vi "test_libssh2_sftp_realpath.vi"() -> ()   [LabVIEW 2013, in "libssh2_integration_tests.lvlib"]
uses:
  libssh2_integration_tests.lvlib
  <vilib>/addons/_JKI Toolkits/Caraya/classes/Test/Test.lvclass
  libssh2/libssh2.lvlib
  <vilib>/addons/_JKI Toolkits/Caraya/classes/Assert/Assert.lvclass
panel:
  out "error out":errorcluster
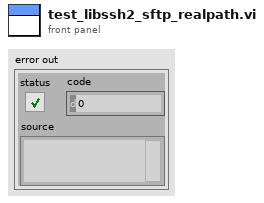
[diagram p1: front panel]
types:
  T1 = typedef "libssh2.lvlib/Session Refnum.ctl" = refnum<k1>
  T2 = typedef "libssh2.lvlib/SFTP Refnum.ctl" = refnum<k1>
  T3 = typedef "libssh2.lvlib/SFTP Handle Refnum.ctl" = refnum<k1>
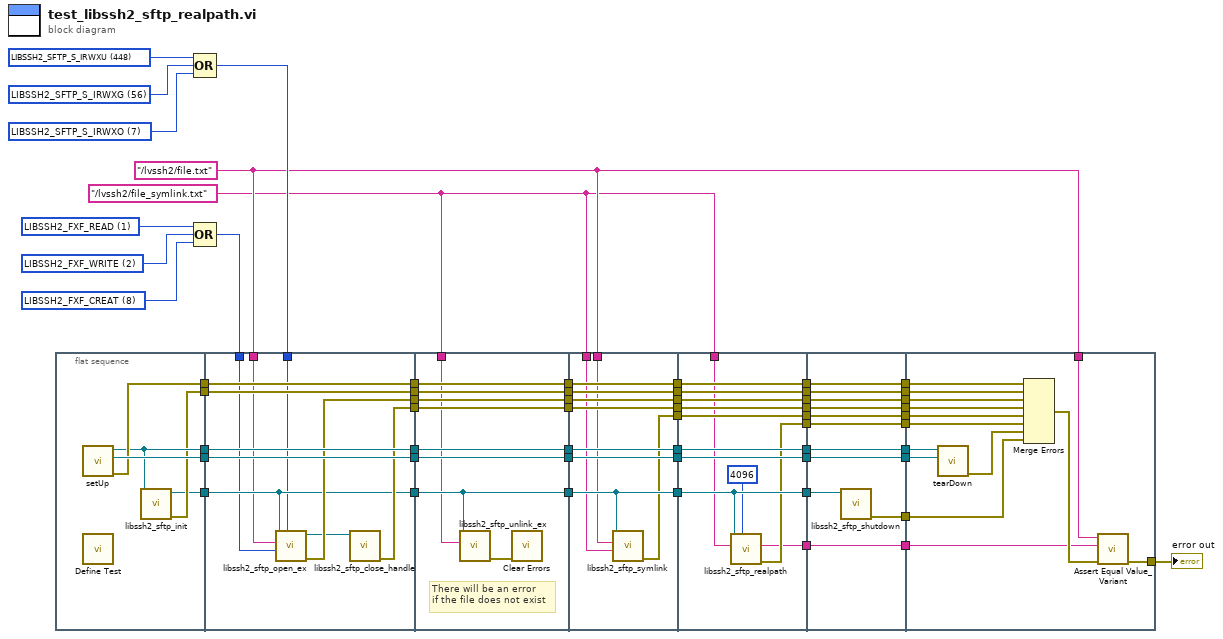
[diagram p0: block diagram]
diagram:
  w1 = "/lvssh2/file_symlink.txt" ("filename")
  w47 = u32 2 items=["LIBSSH2_FXF_READ"=1, "LIBSSH2_FXF_WRITE"=2, "LIBSSH2_FXF_APPEND"=4, "LIBSSH2_FXF_CREAT"=8, "LIBSSH2_FXF_TRUNC"=16, "LIBSSH2_FXF_EXCL"=32] ("flags")
  w48 = u32 1 items=["LIBSSH2_FXF_READ"=1, "LIBSSH2_FXF_WRITE"=2, "LIBSSH2_FXF_APPEND"=4, "LIBSSH2_FXF_CREAT"=8, "LIBSSH2_FXF_TRUNC"=16, "LIBSSH2_FXF_EXCL"=32] ("flags")
  w46 = u32 8 items=["LIBSSH2_FXF_READ"=1, "LIBSSH2_FXF_WRITE"=2, "LIBSSH2_FXF_APPEND"=4, "LIBSSH2_FXF_CREAT"=8, "LIBSSH2_FXF_TRUNC"=16, "LIBSSH2_FXF_EXCL"=32] ("flags")
  w16 = "/lvssh2/file.txt" ("filename")
  w50 = 7 items=["LIBSSH2_SFTP_S_IRWXU"=448, "LIBSSH2_SFTP_S_IRUSR"=256, "LIBSSH2_SFTP_S_IWUSR"=128, "LIBSSH2_SFTP_S_IXUSR"=64, "LIBSSH2_SFTP_S_IRWXG"=56, "LIBSSH2_SFTP_S_IRGRP"=32, "LIBSSH2_SFTP_S_IWGRP"=16, "LIBSSH2_SFTP_S_IXGRP"=8, "LIBSSH2_SFTP_S_IRWXO"=7, "LIBSSH2_SFTP_S_IROTH"=4, "LIBSSH2_SFTP_S_IWOTH"=2, "LIBSSH2_SFTP_S_IXOTH"=1] ("mode")
  w51 = 56 items=["LIBSSH2_SFTP_S_IRWXU"=448, "LIBSSH2_SFTP_S_IRUSR"=256, "LIBSSH2_SFTP_S_IWUSR"=128, "LIBSSH2_SFTP_S_IXUSR"=64, "LIBSSH2_SFTP_S_IRWXG"=56, "LIBSSH2_SFTP_S_IRGRP"=32, "LIBSSH2_SFTP_S_IWGRP"=16, "LIBSSH2_SFTP_S_IXGRP"=8, "LIBSSH2_SFTP_S_IRWXO"=7, "LIBSSH2_SFTP_S_IROTH"=4, "LIBSSH2_SFTP_S_IWOTH"=2, "LIBSSH2_SFTP_S_IXOTH"=1] ("mode")
  w52 = 448 items=["LIBSSH2_SFTP_S_IRWXU"=448, "LIBSSH2_SFTP_S_IRUSR"=256, "LIBSSH2_SFTP_S_IWUSR"=128, "LIBSSH2_SFTP_S_IXUSR"=64, "LIBSSH2_SFTP_S_IRWXG"=56, "LIBSSH2_SFTP_S_IRGRP"=32, "LIBSSH2_SFTP_S_IWGRP"=16, "LIBSSH2_SFTP_S_IXGRP"=8, "LIBSSH2_SFTP_S_IRWXO"=7, "LIBSSH2_SFTP_S_IROTH"=4, "LIBSSH2_SFTP_S_IWOTH"=2, "LIBSSH2_SFTP_S_IXOTH"=1] ("mode")
  n1 = flat-sequence {
    tunnel: [w61] -> w58
    tunnel: [w63] -> w57
    tunnel: [w62] -> w56
    tunnel: [w60] -> w54
    tunnel: [w59] -> w53
    tunnel: [w74] -> w15
    tunnel: [w73] -> w13
    tunnel: [w68] -> w11
    tunnel: [w72] -> w9
    tunnel: [w71] -> w7
    tunnel: [w70] -> w5
    tunnel: [w69] -> w3
    tunnel: w45 -> [w65]
    tunnel: w16 -> [w66]
    tunnel: w49 -> [w67]
    tunnel: w53 -> [w68]
    tunnel: w54 -> [w71]
    tunnel: w56 -> [w72]
    tunnel: w57 -> [w73]
    tunnel: w58 -> [w74]
    tunnel: w15 -> [w83]
    tunnel: [w83] -> w14
    tunnel: w13 -> [w82]
    tunnel: [w82] -> w12
    tunnel: w11 -> [w76]
    tunnel: [w76] -> w10
    tunnel: w9 -> [w81]
    tunnel: [w81] -> w8
    tunnel: w7 -> [w80]
    tunnel: [w80] -> w6
    tunnel: w5 -> [w79]
    tunnel: [w79] -> w4
    tunnel: w3 -> [w78]
    tunnel: [w78] -> w2
    tunnel: w1 -> [w75]
    tunnel: w14 -> [w93]
    tunnel: [w93] -> w36
    tunnel: w12 -> [w92]
    tunnel: [w92] -> w34
    tunnel: w10 -> [w89]
    tunnel: [w89] -> w32
    tunnel: w8 -> [w91]
    tunnel: [w91] -> w29
    tunnel: w6 -> [w90]
    tunnel: [w90] -> w27
    tunnel: w16 -> [w85]
    tunnel: w1 -> [w86]
    tunnel: w4 -> [w88]
    tunnel: [w88] -> w25
    tunnel: w2 -> [w87]
    tunnel: [w87] -> w23
    tunnel: [w84] -> w21
    tunnel: w36 -> [w105]
    tunnel: [w105] -> w35
    tunnel: w34 -> [w104]
    tunnel: [w104] -> w33
    tunnel: w32 -> [w98]
    tunnel: [w98] -> w31
    tunnel: [w95] -> w30
    tunnel: w29 -> [w103]
    tunnel: [w103] -> w28
    tunnel: w27 -> [w102]
    tunnel: [w102] -> w26
    tunnel: w25 -> [w101]
    tunnel: [w101] -> w24
    tunnel: w23 -> [w100]
    tunnel: [w100] -> w22
    tunnel: w21 -> [w99]
    tunnel: [w99] -> w20
    tunnel: w1 -> [w97]
    tunnel: [w96] -> w18
    tunnel: w35 -> [w116]
    tunnel: [w116] -> w44
    tunnel: w33 -> [w115]
    tunnel: [w115] -> w43
    tunnel: w31 -> [w111]
    tunnel: w30 -> [w114]
    tunnel: [w114] -> w42
    tunnel: w28 -> [w113]
    tunnel: [w113] -> w41
    tunnel: w26 -> [w112]
    tunnel: [w112] -> w40
    tunnel: [w110] -> w39
    tunnel: w24 -> [w109]
    tunnel: [w109] -> w38
    tunnel: w22 -> [w108]
    tunnel: [w108] -> w37
    tunnel: w20 -> [w107]
    tunnel: [w107] -> w19
    tunnel: w18 -> [w106]
    tunnel: [w106] -> w17
    tunnel: w44 -> [w130]
    tunnel: w43 -> [w129]
    tunnel: w42 -> [w118]
    tunnel: w41 -> [w128]
    tunnel: [w125] -> w55
    tunnel: w40 -> [w124]
    tunnel: w39 -> [w123]
    tunnel: w38 -> [w122]
    tunnel: w37 -> [w121]
    tunnel: w19 -> [w120]
    tunnel: w17 -> [w119]
    tunnel: w16 -> [w117]
    frame #0 {
      n2 = call "setUp.vi"() -> ("error out"=w62:errorcluster, "connection ID"=w63:refnum<k5>, "session"=w61:T1)  [unwired: 9 in]
      n3 = call <vilib>:"Define Test.vi"() -> ()  [unwired: 10 in, 2 out]
      n4 = call "libssh2_sftp_init.vi"("session"=w61) -> ("error out"=w60:errorcluster, "sftp"=w59:T2)  [unwired: 9 in]
    }
    frame #1 {
      n5 = call "libssh2_sftp_open_ex.vi"("mode"=w67, "flags"=w65, "filename"=w66, "sftp"=w68) -> ("error out"=w70:errorcluster, "sftp handle"=w64:T3)  [unwired: 6 in]
      n6 = call "libssh2_sftp_close_handle.vi"("sftp handle"=w64) -> ("error out"=w69:errorcluster)  [unwired: 10 in]
    }
    frame #2 {
      # "There will be an error\nif the file does not exist"
      n7 = call "libssh2_sftp_unlink_ex.vi"("file"=w75, "sftp"=w76) -> ("error out"=w77:errorcluster)  [unwired: 9 in]
      n8 = call <vilib>:"Clear Errors.vi"("error in (no error)"=w77) -> ()  [unwired: 6 in, 1 out]
    }
    frame #3 {
      n9 = call "libssh2_sftp_symlink.vi"("target"=w86, "path"=w85, "sftp"=w89) -> ("error out"=w84:errorcluster)  [unwired: 8 in]
    }
    frame #4 {
      n10 = call "libssh2_sftp_realpath.vi"("maxlen"=u32 4096, "path"=w97, "sftp"=w98) -> ("error out"=w96:errorcluster, "target"=w95:string)  [unwired: 7 in]
    }
    frame #5 {
      n11 = call "libssh2_sftp_shutdown.vi"("sftp"=w111) -> ("error out"=w110:errorcluster)  [unwired: 10 in]
    }
    frame #6 {
      n12 = call "tearDown.vi"("connection ID"=w129, "session"=w130) -> ("error out"=w127:errorcluster)  [unwired: 9 in]
      n13 = Merge Errors(w128, w124, w122, w121, w120, w119, w127, w123) -> (w126:errorcluster)
      n14 = call <vilib>:"Assert Equal Value_Variant.vi"("error in (no error)"=w126, "Y"=w118, "X"=w117) -> ("error out"=w125:errorcluster)  [unwired: 7 in, 1 out]
    }
  }
  n15 = Compound Arithmetic op=OR(w52, w51, w50) -> (w49:i32)
  n16 = Compound Arithmetic op=OR(w48, w47, w46) -> (w45:u32)
  "error out" <- w55
